vi "Send message to initialize all modules.vi"(10 "System config file path":path, 11 "Messenger referencies":T1) -> ()   [LabVIEW 2022 SP3]
doc: "Sends initialization messages to all modules. System configuration file path is send as data."
uses:
  Subsystem modules/Messenger service/Data types/Messenger referencies.ctl
  Subsystem modules/Magnet module/ctl/MSG to magnet.ctl
  Subsystem modules/Magnet module/ctl/Magnet Orders.ctl
  Subsystem modules/Servo drive module/ctl/Servo MSG.ctl
  Subsystem modules/Servo drive module/ctl/Servo commands.ctl
  Subsystem modules/Lock-in module/ctl/MFLI_message for module.ctl
  Subsystem modules/Lock-in module/ctl/MFLI_command enum.ctl
  Subsystem modules/Sample rotator/ctl/MSG to Rotator.ctl
  Subsystem modules/Sample rotator/ctl/Rotator commands.ctl
  Subsystem modules/THz module/ctl/THz Message for module.ctl
  Subsystem modules/THz module/ctl/THz commands enum.ctl
  Subsystem modules/THz module/ctl/VDI config constants.ctl
  Subsystem modules/THz module/ctl/Synth configs.ctl
  Subsystem modules/Temperature control module/ctl/MSG for VTI.ctl
  Subsystem modules/Temperature control module/ctl/TC commands.ctl
  Subsystem modules/Magnet module/Magnet module.lvlib
  Subsystem modules/Servo drive module/Servo drive module.lvlib
  Subsystem modules/Lock-in module/Lock-in module.lvlib
  Subsystem modules/Sample rotator/SampleRotator.lvlib
  Subsystem modules/THz module/THz source modeule.lvlib
  Subsystem modules/Temperature control module/Temperature controller.lvlib
  Subsystem modules/Messenger service/MessengerLib.lvlib
panel:
  out "error out":errorcluster
  in  "error in (no error)":errorcluster
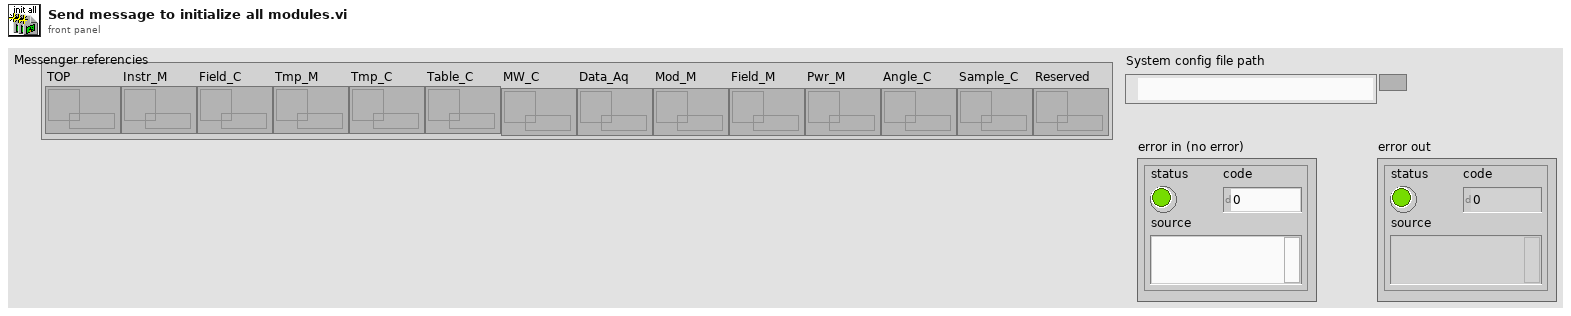
[diagram p1: front panel]
types:
  T1 = typedef "MessengerLib.lvlib/Messenger referencies.ctl" = cluster{"TOP":refnum<queue>, "Instr_M":refnum<queue>, "Field_C":refnum<queue>, "Tmp_M":refnum<queue>, "Tmp_C":refnum<queue>, "Table_C":refnum<queue>, "MW_C":refnum<queue>, "Data_Aq":refnum<queue>, "Mod_M":refnum<queue>, "Field_M":refnum<queue>, "Pwr_M":refnum<queue>, "Angle_C":refnum<queue>, "Sample_C":refnum<queue>, "Reserved":refnum<queue>}
  T2 = typedef "Temperature controller.lvlib/TC commands.ctl" = enum16{"Initialize", "Update", "Stop tmp change", "Set temperature", "Set point", "Disconnect", "End", "Ignore"}
  T3 = typedef "Temperature controller.lvlib/MSG for VTI.ctl" = cluster{"Command":T2, "Data":variant}
  T4 = typedef "Lock-in module.lvlib/MFLI_command enum.ctl" = enum16{"Initialize", "Update", "Set parameters", "Set module", "Set individual parameters", "Get point", "Get array", "Disconnect", "End", "Ignore"}
  T5 = typedef "THz source modeule.lvlib/VDI config constants.ctl" = cluster{"Master":T6, "Follower":T6}
  T6 = typedef "THz source modeule.lvlib/Synth configs.ctl" = cluster{"Lower limit [GHz]":dbl, "Upper limit [GHz]":dbl, "Name":string, "Handle":string, "Description":string}
  T7 = typedef "THz source modeule.lvlib/THz commands enum.ctl" = enum16{"Ignore", "Connect", "Update", "Set parameters", "Disconnect", "End"}
  T8 = typedef "SampleRotator.lvlib/Rotator commands.ctl" = enum16{"Ignore", "Initialize", "Update", "Set parameters", "Stop movement", "Set position", "Disconnect", "End"}
  T9 = typedef "THz source modeule.lvlib/THz Message for module.ctl" = cluster{"Command":T7, "Data":variant}
  T10 = typedef "SampleRotator.lvlib/MSG to Rotator.ctl" = cluster{"Command":T8, "Data":variant}
  T11 = typedef "Lock-in module.lvlib/MFLI_message for module.ctl" = cluster{"Command":T4, "Data":variant}
  T12 = typedef "Magnet module.lvlib/Magnet Orders.ctl" = enum16{"Ignore", "Connect", "Update", "Switch mode", "Set field", "Stop ramping", "Equalize output", "Zero output", "Flip polarity", "Blackout", "Set timer", "Eval temperatures", "Disconnect"}
  T13 = typedef "Servo drive module.lvlib/Servo commands.ctl" = enum16{"Initialize", "Update", "Move by", "Move to", "Stop", "Ignore", "Disconnect", "End"}
  T14 = typedef "Servo drive module.lvlib/Servo MSG.ctl" = cluster{"Command":T13, "Data":variant}
  T15 = typedef "Magnet module.lvlib/MSG to magnet.ctl" = cluster{"Command":T12, "Data":variant}
  T16 = typedef "Magnet module.lvlib/Magnet config constants.ctl" = cluster{"Switch resistant [K]":dbl, "Switch superconducting [K]":dbl, "First stage critical temperature [K]":dbl, "Second stage critical temperature [K]":dbl, "Inner magnet critical temperature [K]":dbl, "Outer magnet critical temperature [K]":dbl, "Field Constant [T/A]":dbl, "Maximum Current [A]":dbl, "Maximum field [T]":dbl, "Maximum source ramp [A/s]":dbl, "Source precision [T]":dbl, "Ramp limits [A/s]":dbl[], "Field limits [T]":dbl[], "SMS":refnum<visa-resource-name>, "LSC218":refnum<visa-resource-name>}
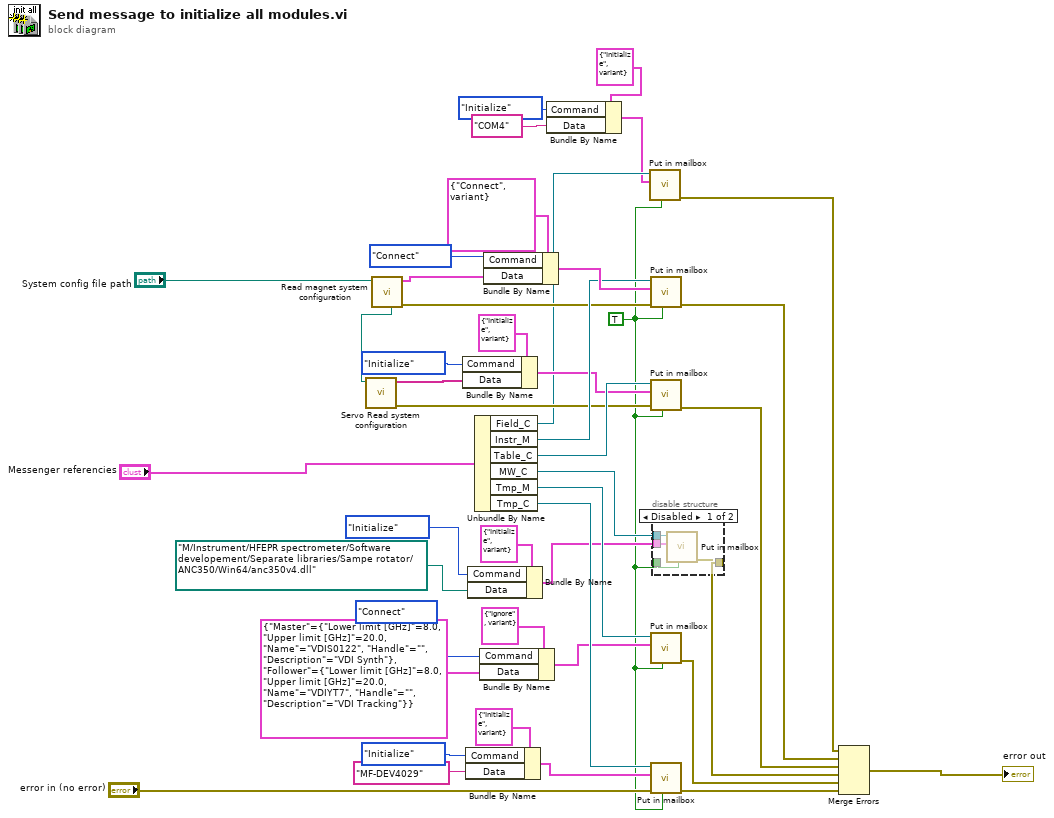
[diagram p0: block diagram]
diagram:
  w2 = TRUE
  n1 = call "Read magnet system configuration.vi"("MAG config file path"="System config file path") -> ("error out"=w9:errorcluster, "Magnet Constantsout"=w25:T16, "file path out"=w10:path)  [unwired: 8 in]
  n2 = call "Servo Read system configuration.vi"("MAG config file path"=w10) -> ("error out"=w8:errorcluster, "IP addresses"=w12:string[])  [unwired: 8 in, 1 out]
  n3 = Bundle By Name(cluster=T14 {"Command"=enum."Initialize", "Data"=variant(dbl[] [])} ("MSG to Servo"), "Command"=Servo_commands."Initialize", "Data"=w12) -> (w26:T14)
  n4 = Bundle By Name(cluster=T11 {"Command"=enum."Initialize", "Data"=variant} ("MSG for  ACQ"), "Command"=MFLI_command_enum."Initialize", "Data"="MF-DEV4029") -> (w18:T11)
  n5 = Bundle By Name(cluster=T10 {"Command"=enum."Initialize", "Data"=variant} ("MSG to rotator"), "Command"=Rotator_commands."Initialize", "Data"=path "M:/Instrument/HFEPR spectrometer/Software developement/Separate libraries/Sampe rotator/ANC350/Win64/anc350v4.dll" ("File Path Control")) -> (w22:T10)
  n6 = Unbundle By Name("Messenger referencies") -> ("Field_C"=w7:refnum<queue>, "Instr_M"=w41:refnum<queue>, "Table_C"=w40:refnum<queue>, "MW_C"=w39:refnum<queue>, "Tmp_M"=w38:refnum<queue>, "Tmp_C"=w37:refnum<queue>)
  n7 = Bundle By Name(cluster=T9 {"Command"=enum."Ignore", "Data"=variant} ("Incoming msg"), "Command"=THz_commands_enum."Connect", "Data"=T5 {"Master"={"Lower limit [GHz]"=8.0, "Upper limit [GHz]"=20.0, "Name"="VDIS0122", "Handle"="", "Description"="VDI Synth"}, "Follower"={"Lower limit [GHz]"=8.0, "Upper limit [GHz]"=20.0, "Name"="VDIYT7", "Handle"="", "Description"="VDI Tracking"}} ("VDI config constants")) -> (w19:T9)
  n8 = Bundle By Name(cluster=T15 {"Command"=enum."Connect", "Data"=variant(enum16{"Ramping", "Perzistant"} enum."Ramping")} ("MSG to magnet"), "Command"=Magnet_Orders."Connect" ("Order"), "Data"=w25) -> (w42:T15)
  n9 = Bundle By Name(cluster=T3 {"Command"=enum."Initialize", "Data"=variant} ("MSG for VTI"), "Command"=TC_commands."Initialize", "Data"="COM4") -> (w6:T3)
  n10 = call "Put in mailbox.vi"("Priority? (F)"=w2, "Message"=w6, "Queue in"=w7) -> ("error out"=w3:errorcluster)  [unwired: 6 in, 2 out]
  n11 = call "Put in mailbox.vi"("Priority? (F)"=w2, "error in (no error)"=w9, "Message"=w42, "Queue in"=w41) -> ("error out"=w32:errorcluster)  [unwired: 5 in, 2 out]
  n12 = call "Put in mailbox.vi"("Priority? (F)"=w2, "error in (no error)"=w8, "Message"=w26, "Queue in"=w40) -> ("error out"=w33:errorcluster)  [unwired: 5 in, 2 out]
  n13 = call "Put in mailbox.vi"("Priority? (F)"=w2, "Message"=w19, "Queue in"=w38) -> ("error out"=w35:errorcluster)  [unwired: 6 in, 2 out]
  n14 = call "Put in mailbox.vi"("Priority? (F)"=w2, "error in (no error)"="error in (no error)", "Message"=w18, "Queue in"=w37) -> ("error out"=w36:errorcluster)  [unwired: 5 in, 2 out]
  n15 = disable-structure shown="Disabled" {
    disable-tunnel: w39 -> [w48 _]
    disable-tunnel: [w47 _] -> w34
    disable-tunnel: w22 -> [w46 _]
    disable-tunnel: w2 -> [w45 _]
    frame Disabled {
      n16 = call "Put in mailbox.vi"("Priority? (F)"=w45, "Message"=w46, "Queue in"=w48) -> ("error out"=w47:errorcluster)  [unwired: 6 in, 2 out]
    }
    frame Enabled {
    }
  }
  n17 = Merge Errors(w3, w32, w33, w34, w35, w36) -> (→"error out":errorcluster)
